vi "QTrkFindBeads.vi"(0 "Image":T1, 5 "Sample corner pos":cluster{"X":i32, "Y":i32}, 7 "roi":i32=60, 9 "Minimum correlation [0-1]":sgl=0.6, 11 "Distance between beads\n(relative to ROI)":sgl=0.7) -> (4 "Bead positions":cluster{"X":i32, "Y":i32}[](array[cluster]))   [LabVIEW 2011]
uses:
  <vilib>/vision/Image Controls.llb/IMAQ Image.ctl
  QTrkDLL.vi
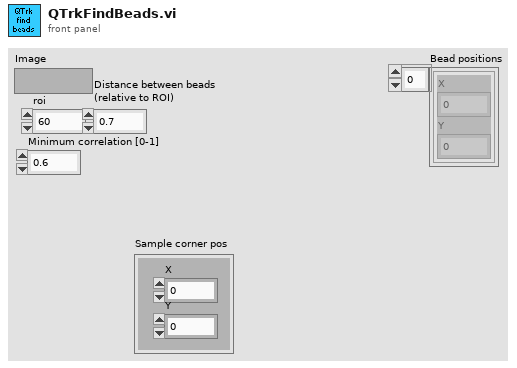
[diagram p1: front panel]
types:
  T1 = typedef "IMAQ Image.ctl" = refnum<image>
  T2 = enum32{"Map Pixel Pointer", "Unmap Pixel Pointer", "Get Pixels Infos"}
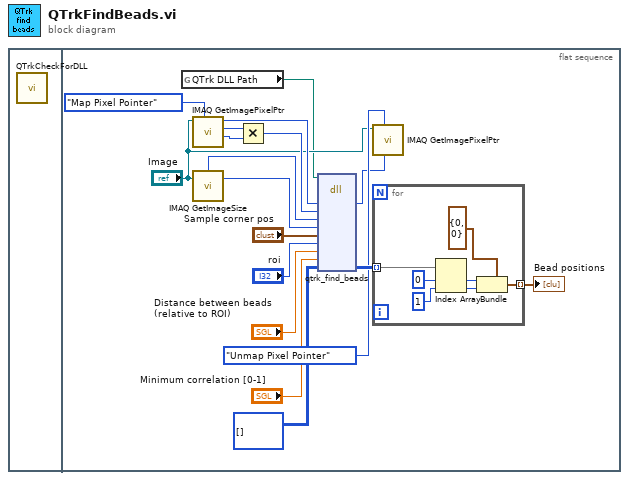
[diagram p0: block diagram]
diagram:
  n1 = flat-sequence {
    frame #0 {
      n2 = call "QTrkCheckForDLL.vi"() -> ()  [unwired: 12 in]
    }
    frame #1 {
      n3 = global read "QTrkDLL.vi" "QTrk DLL Path"() -> (w1:path)
      n4 = call "IMAQ GetImagePixelPtr"("Function"=T2."Map Pixel Pointer", "Image"="Image") -> ("Pixel Size (Bytes)"=w17:i32, "LineWidth(Pixels)"=w16:i32, "Pixel Pointer out"=w9:u64)  [unwired: 4 in, 3 out]
      n5 = call "IMAQ GetImageSize"("Image"="Image") -> ("Y Resolution"=w4:i32, "X Resolution"=w5:i32)  [unwired: 3 in, 1 out]
      n6 = Multiply(x=w16, y=w17) -> (x*y=w10:i32)
      n7 = dll-call lib="D:/jcnossen1/qtrk/qtrk/lv/qtrk-labview.dll" fn="qtrk_find_beads"(path in=w1, "image"=w9, "pitch"=w10, "w"=w5, "h"=w4, "smpCornerPos"="Sample corner pos", "roi"="roi", "imgRelDistance"="Distance between beads\n(relative to ROI)", "acceptance"="Minimum correlation [0-1]", "output"=i32[][] []) -> ("image"=w7:u64, "output"=w12:i32[][])  [unwired: 10 in, 2 out]
      n8 = call "IMAQ GetImagePixelPtr"("Pixel Pointer in"=w7, "Function"=T2."Unmap Pixel Pointer", "Image"="Image") -> ()  [unwired: 3 in, 6 out]
      n9 = for {
        tunnel: w12 -> [w24] mode=indexing
        tunnel: [w19] -> w11 mode=indexing
        n10 = Index Array(array=w24, index #1=0 ("index"), index #2=1 ("index")) -> (element #1=w21:i32, element #2=w20:i32)
        n11 = Bundle(cluster=cluster{"X":i32, "Y":i32} {"X"=0, "Y"=0} ("Sample corner pos 2"), "X"=w21, "Y"=w20) -> (w19:cluster{"X":i32, "Y":i32})
      }
      "Bead positions" <- w11
    }
  }
